vi "delete from sorted list.vi"(10 "element to delete":string, 11 "sorted list in":T1) -> (1 "deleted index":i32, 2 "success?":bool, 3 "sorted list out":T1)   [LabVIEW 2013, in "tag bus.lvlib" / "binary search.lvlib"]
doc: "Removes a single element from a sorted list."
uses:
  binary search.lvlib
  sorted list.ctl
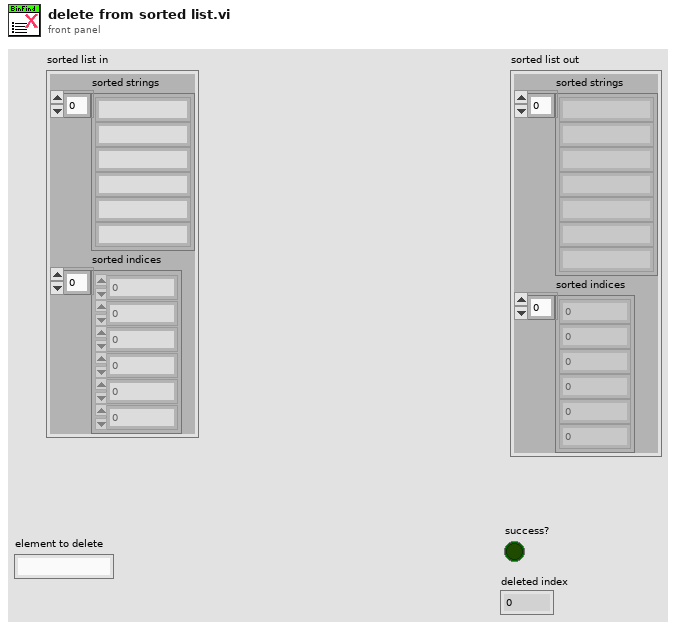
[diagram p1: front panel]
types:
  T1 = typedef "tag bus.lvlib/binary search.lvlib/sorted list.ctl" = cluster{"sorted strings":string[], "sorted indices":i32[]}
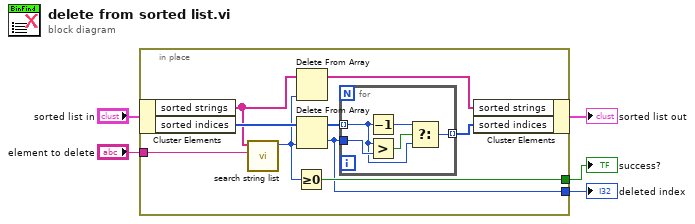
[diagram p0: block diagram]
diagram:
  n1 = in-place {
    in-place-border: "element to delete" -> [w10]
    in-place-border: [w14] -> w2
    in-place-border: [w7] -> w1
    n2 = in-place-cluster #1("sorted list in") -> ("sorted strings"=w11:string[], "sorted indices"=w13:i32[])
    n3 = call "search string list.vi"("string to locate"=w10, "sorted strings"=w11) -> ("index"=w9:i32)  [unwired: 9 in]
    n4 = Greater Or Equal To 0?(x=w9) -> (x >= 0?=w14:bool)
    n5 = Delete From Array(array=w11, index=w9) -> (array with subset deleted=w12:string[])  [unwired: 1 in, 1 out]
    n6 = Delete From Array(array=w13, index=w9) -> (deleted portion=w7:i32, array with subset deleted=w8:i32[])  [unwired: 1 in]
    n7 = for {
      tunnel: w8 -> [w16] mode=indexing
      tunnel: w7 -> [w19]
      tunnel: [w15] -> w6 mode=indexing
      n8 = Decrement(x=w16) -> (x-1=w17:i32)
      n9 = Greater?(x=w16, y=w19) -> (0:w18:bool)
      n10 = Select(t=w17, s=w18, f=w16) -> (s? t:f=w15:i32)
    }
    n11 = in-place-cluster #1("sorted strings"=w12, "sorted indices"=w6) -> (→"sorted list out":T1)
  }
  "success?" <- w2
  "deleted index" <- w1
